vi "Unpack 32I12's Packed into 24xI16 as 32xI16 Poly.vi"   [LabVIEW 2012]
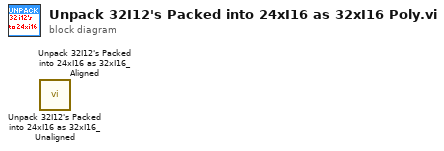
[diagram p0: block diagram]
diagram:
  n1 = call <userlib>:"Unpack 32I12's Packed into 24xI16 as 32xI16_Unaligned.vi"() -> ()  [unwired: 10 in, 2 out]
  n2 = call <userlib>:"Unpack 32I12's Packed into 24xI16 as 32xI16_Aligned.vi"() -> ()  [unwired: 10 in, 2 out]
